vi "Update Configuration MCL.vi"(5 "number of RTD input channels":i32=8, 6 "error in":errorcluster, 7 "_9216 Config":T1={"Conversion Time"=0, "Degree Range"=[], "RTD_Type"=[1], "RTD_A"=[], "RTD_B"=[], "RTD_C"=[], "RTD_Ro"=[]} {"RTD_Type" items=["TCR3851"=1, "TCR3750"=2, "TCR3916"=3, "TCR3920"=4, "TCR3911"=5, "TCR3928"=6, "Custom"=0]; "Degree Range" items=["Raw Ohms", "Degrees Kelvin", "Degrees Celsius", "Degrees Fahrenheit", "Degrees Rankine"]; "Conversion Time" items=["200 ms", "2.5 ms"]}, 9 "_Channel Refnum":refnum<vi>) -> (0 "error out":errorcluster)   [LabVIEW 2020, in "Modules.lvlib" / "9216.lvclass"]
uses:
  9216.lvclass
panel:
  in  "RTD Type":u8(ring) items=["TCR3851"=1, "TCR3750"=2, "TCR3916"=3, "TCR3920"=4, "TCR3911"=5, "TCR3928"=6, "Custom"=0]
  in  "Degree Range":u8(ring) items=["Raw Ohms", "Degrees Kelvin", "Degrees Celsius", "Degrees Fahrenheit", "Degrees Rankine"]
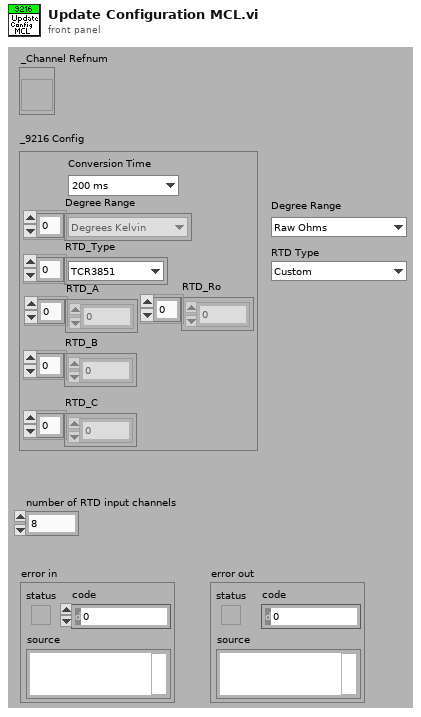
[diagram p1: front panel]
types:
  T1 = cluster{"Conversion Time":u16, "Degree Range":u8[], "RTD_Type":u8[], "RTD_A":dbl[], "RTD_B":dbl[], "RTD_C":dbl[], "RTD_Ro":dbl[]}
  T2 = typedef "LVStringsAndValuesArrayTypeDef_U8.ctl" = cluster{"String":string, "Value":u8}[]
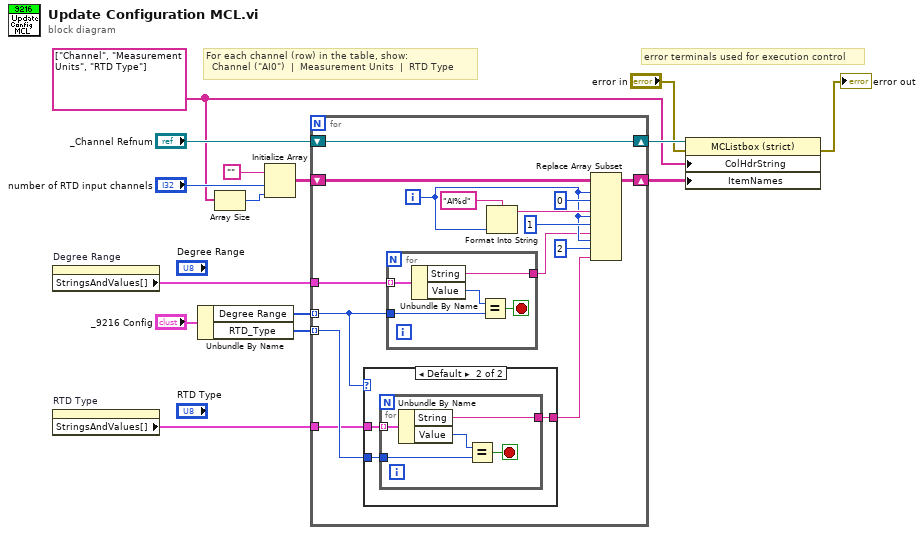
[diagram p0: block diagram]
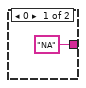
[diagram p2: hidden frame]
diagram:
  w4 = string[] ["Channel", "Measurement Units", "RTD Type"]
  # "For each channel (row) in the table, show:\n  Channel (\"AI0\")  |  Measurement Units  |  RTD Type"
  # "error terminals used for execution control"
  n1 = property on="Degree Range" class="Ring (strict)"() -> ("StringsAndValues[]"=w7:T2)  [unwired: 2 in, 2 out]
  n2 = property on="RTD Type" class="Ring (strict)"() -> ("StringsAndValues[]"=w8:T2)  [unwired: 2 in, 2 out]
  n3 = Unbundle By Name("_9216 Config") -> ("Degree Range"=w6:u8[], "RTD_Type"=w9:u8[])
  n4 = Array Size(array=w4) -> (size(s)=w3:i32)
  n5 = Initialize Array("", "number of RTD input channels", w3) -> (w13:string[][])
  n6 = for {
    shift-right: [w28] -> w5
    shift-left: w13 -> [w27]
    shift-right: [w30] -> w15
    shift-left: "_Channel Refnum" -> [w30]
    tunnel: w9 -> [w20] mode=indexing
    tunnel: w6 -> [w16] mode=indexing
    tunnel: w8 -> [w18]
    tunnel: w7 -> [w17]
    i -> [w23]
    n7 = case shown="Default" w16 {
      tunnel: w20 -> [_ w34]
      tunnel: ["NA" ("Section") w33] -> w19
      tunnel: w18 -> [_ w32]
      frame 0 {
      }
      frame Default {
        n8 = for {
          tunnel: w32 -> [w39] mode=indexing
          tunnel: w34 -> [w37]
          tunnel: [w35] -> w33
          stop <- w36 stop-if-true
          n9 = Unbundle By Name(w39) -> ("String"=w35:string, "Value"=w38:u8)
          n10 = Equal?(x=w38, y=w37) -> (x = y?=w36:bool)
        }
      }
    }
    n11 = for {
      tunnel: w17 -> [w44] mode=indexing
      tunnel: w16 -> [w42]
      tunnel: [w40] -> w21
      stop <- w41 stop-if-true
      n12 = Unbundle By Name(w44) -> ("String"=w40:string, "Value"=w43:u8)
      n13 = Equal?(x=w43, y=w42) -> (x = y?=w41:bool)
    }
    n14 = Format Into String(format string="AI%d", w23) -> (resulting string=w24:string)  [unwired: 2 in, 1 out]
    n15 = Replace Array Subset(array=w27, new element #1=w24, index (row) #1=w23, index (col) #1=0 ("Column 1"), new element #2=w21, index (row) #2=w23, index (col) #2=1 ("Column 1"), new element #3=w19, index (row) #3=w23, index (col) #3=2 ("disabled index (col)")) -> (w28:string[][])
  }
  n16 = property on="Property Node" class="MCListbox (strict)"(reference=w15, error in="error in", "ColHdrString"=w4, "ItemNames"=w5) -> (error out=→"error out":errorcluster)  [unwired: 1 out]
